vi "Find Workspace.vi"(8 "Error In":errorcluster, 10 "Control In":T2, 11 "Workspace In":refnum<class "Current Position.lvclass">) -> (0 "Error Out":errorcluster, 1 "Workspace Out":T1, 2 "Control Out":T2, 3 "Workspace Out":refnum<class "Current Position.lvclass">)   [LabVIEW 2020, in "Current Position.lvclass"]
uses:
  Current Position.lvclass
  Controller/Controllers.ctl
  Controller/I-O/I-O.lvclass
  Controller/Dispenser/Dispenser.lvclass
  C:/Program Files (x86)/Aerotech/A3200/LabVIEW/2010/Bin/Aerotech.A3200.dll
  Program Files (x86)/Aerotech/A3200/LabVIEW/2010/Bin/Aerotech.A3200.dll
  Workspace.ctl
  Controller/Motion/A3200/A3200.lvclass
  Controller/Controller.lvclass
  Fixture.lvclass
panel:
  in  "Workspace":T1
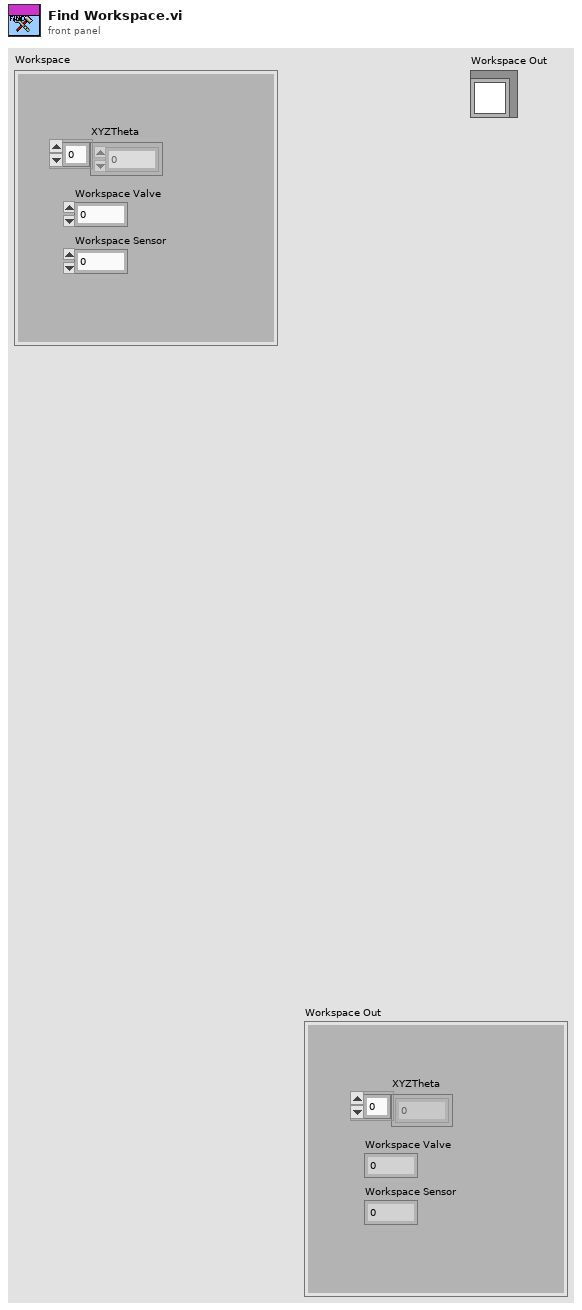
[diagram p1: front panel]
types:
  T1 = typedef "Fixture.lvclass/Workspace.ctl" = cluster{"XYZTheta":dbl[], "Workspace Valve":i32, "Workspace Sensor":i32}
  T2 = typedef "Controller.lvclass/Controllers.ctl" = cluster{"I-O.lvclass":refnum<class "I-O.lvclass">, "Dispenser.lvclass":refnum<class "Dispenser.lvclass">, "Gantry":refnum<k24>}
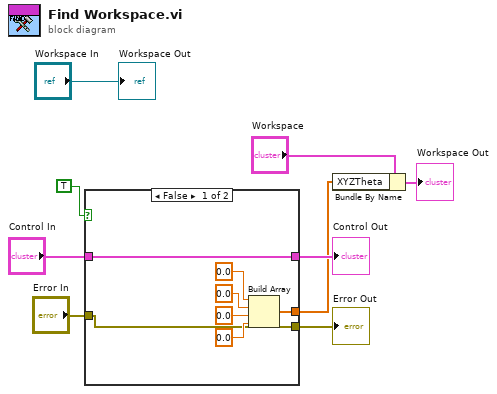
[diagram p0: block diagram]
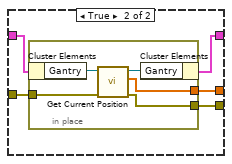
[diagram p2: hidden frame]
diagram:
  n1 = case shown="False" TRUE {
    tunnel: "Control In" -> [w16 w21]
    tunnel: [w16 w20] -> w8
    tunnel: [w15 w19] -> w6
    tunnel: "Error In" -> [w10 w18]
    tunnel: [w10 w17] -> w1
    frame False {
      n2 = Build Array(0.0, 0.0, 0.0, 0.0) -> (w15:dbl[])
    }
    frame True {
      n3 = in-place {
        in-place-border: [w26] -> w19
        in-place-border: w18 -> [w23]
        in-place-border: [w22] -> w17
        n4 = in-place-cluster #1(w21) -> ("Gantry"=w25:refnum<k24>)
        n5 = call "Get Current Position.vi"("error in (no error)"=w23, "Gantry In"=w25) -> ("error out"=w22:errorcluster, "XYZTheta Out"=w26:dbl[], "Gantry Out"=w24:refnum<k24>)  [unwired: 7 in]
        n6 = in-place-cluster #1("Gantry"=w24) -> (w20:T2)
      }
    }
  }
  "Error Out" <- w1
  "Control Out" <- w8
  n7 = Bundle By Name(cluster="Workspace", "XYZTheta"=w6) -> (→"Workspace Out":T1)
  "Workspace Out" <- "Workspace In"
